vi "Drain to AMB verify dialog.vi"(11 "d":i32=101) -> (3 "Drain?":bool)   [LabVIEW 2019]
panel:
  out "Message 2":string
  out "Message":string
  in  "Cancel Drain":bool
  in  "Start Drain":bool
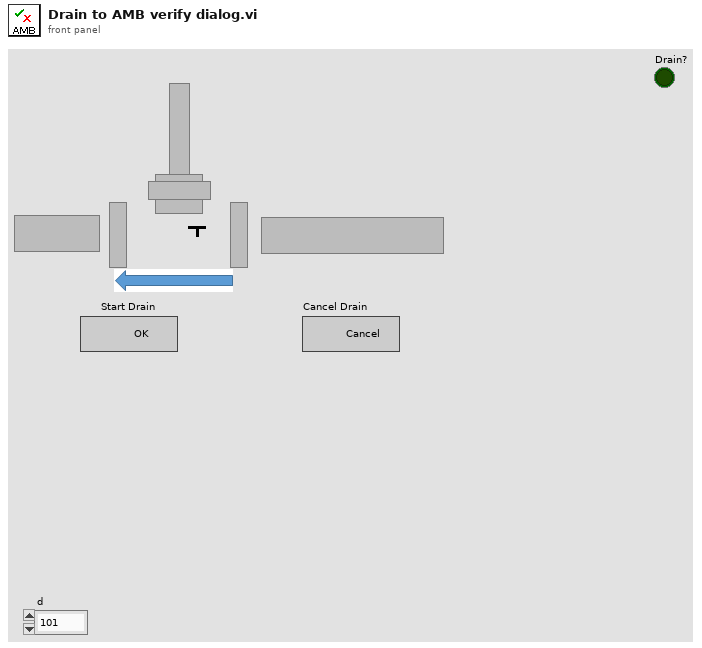
[diagram p1: front panel]
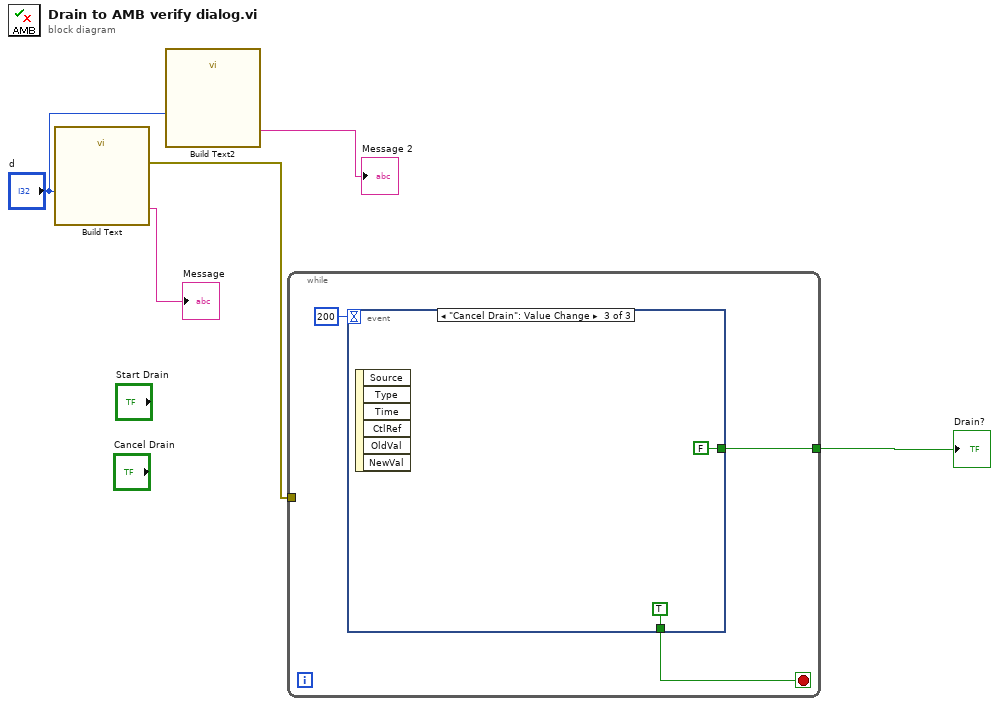
[diagram p0: block diagram]
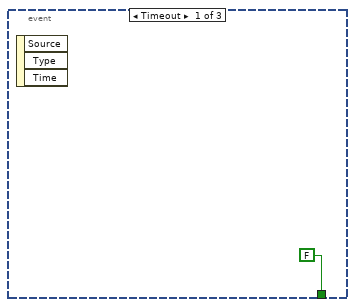
[diagram p2: hidden frame]
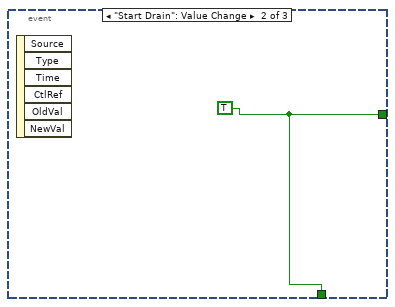
[diagram p3: hidden frame]
diagram:
  n1 = call "Build Text"("d"="d") -> ("Result"=→"Message":string, "error out"=w3:errorcluster)  [unwired: 13 in]
  n2 = call "Build Text2"("d"="d") -> ("Result"=→"Message 2":string)  [unwired: 13 in, 1 out]
  n3 = while {
    tunnel: [w7] -> w5
    tunnel: w3 -> [_]
    stop <- w6 stop-if-true
    n4 = event shown="[2] \"Cancel Drain\": Value Change" {
      selector: _ -> [_ _ _]
      dyn-events: _ -> [_ _ _]
      timeout: 200 -> [_ _ _]
      tunnel: [_ w10 FALSE] -> w7
      tunnel: [FALSE w10 TRUE] -> w6
      event Timeout {
        n5 = event-data() -> ()  [unwired: 1 in, 3 out]
      }
      event "Start Drain": Value Change {
        w10 = TRUE
        n6 = event-data() -> ()  [unwired: 1 in, 6 out]
      }
      event "Cancel Drain": Value Change {
        n7 = event-data() -> ()  [unwired: 1 in, 6 out]
      }
    }
  }
  "Drain?" <- w5
